vi "Call Algorithm.vi"(6 "Backend engine":T1, 8 "error in":errorcluster, 11 "Algorithm ID":string) -> (0 "error out":errorcluster)   [LabVIEW 2013, in "QWTBLVLib.lvlib"]
doc: "Call selected algorithm on previously stored input data and calculation setting."
uses:
  QWTBLVLib.lvlib
  TD Backend Engine.ctl
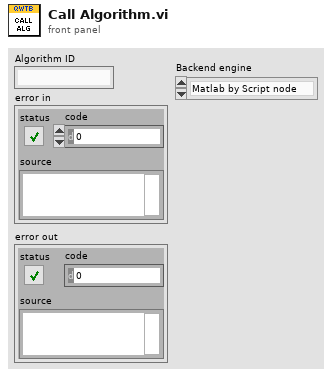
[diagram p1: front panel]
types:
  T1 = typedef "QWTBLVLib.lvlib/TD Backend Engine.ctl" = enum16{"Matlab by Script node", "GNU Octave by GOLPI"}
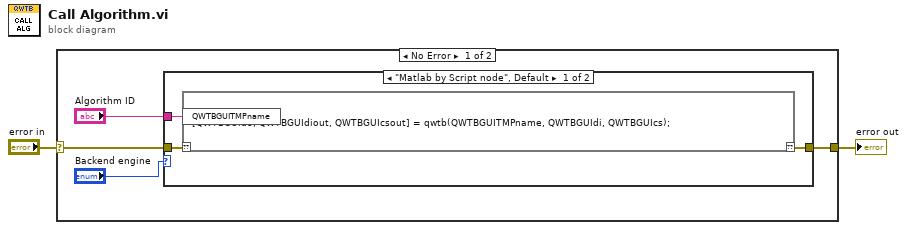
[diagram p0: block diagram]
diagram:
  n1 = case shown="No Error" "error in" {
    selector: "error in" -> [w6 w11]
    tunnel: [w4 w11] -> w2
    frame No Error {
      n2 = case shown="\"Matlab by Script node\", Default" "Backend engine" {
        tunnel: w6 -> [w9 w10]
        tunnel: "Algorithm ID" -> [w8 _]
        tunnel: [w7 w10] -> w4
        frame "Matlab by Script node", Default {
          n3 = script code="[QWTBGUIdo, QWTBGUIdiout, QWTBGUIcsout] = qwtb(QWTBGUITMPname, QWTBGUIdi, QWTBGUIcs);"("??"=w9, "QWTBGUITMPname"=w8) -> ("??"=w7:errorcluster)
        }
        frame "GNU Octave by GOLPI" {
          # "#2do"
        }
      }
    }
    frame Error {
    }
  }
  "error out" <- w2
